vi "Read Log record configuration.vi"(8 "error in (no error)":errorcluster, 11 "Log Record in":refnum<class "Log Record.lvclass">) -> (0 "error out":errorcluster, 2 "Configuration":T1={"OSF node  ID"="", "Conection timeout"=60.0, "Station"="", "Log server "="magx", "Upload to OSF"=FALSE, "Append to lab book"=FALSE, "Filing modules"=["Monitor Controller", "Pulse Controller"]} {"Conection timeout" format="%#_6ps"}, 3 "Log Record out":refnum<class "Log Record.lvclass">)   [LabVIEW 2021, in "Log Record.lvclass"]
uses:
  Log Record.lvclass
  C:/GitHub/LabActor/Template Module/Template Module.lvclass
  Log Record Configuration.ctl
  Template Module/Template Module.lvclass/Template Module.ctl
  Template Module/Read Configuration.vi
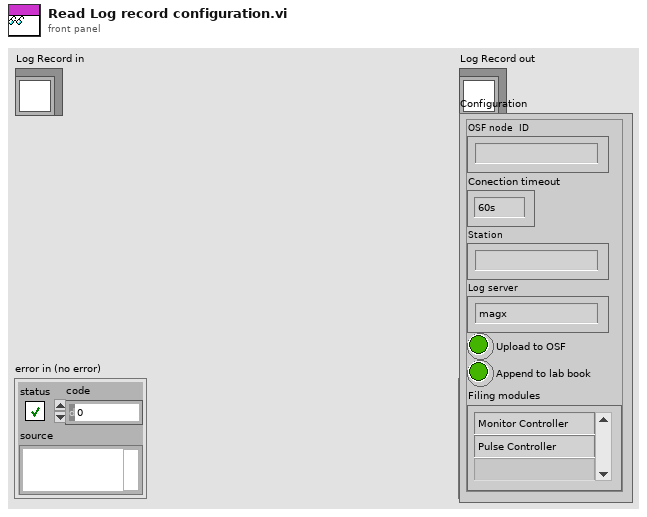
[diagram p1: front panel]
types:
  T1 = typedef "Log Record Configuration.ctl" = cluster{"OSF node  ID":string, "Conection timeout":dbl, "Station":string, "Log server ":string, "Upload to OSF":bool, "Append to lab book":bool, "Filing modules":string[]}
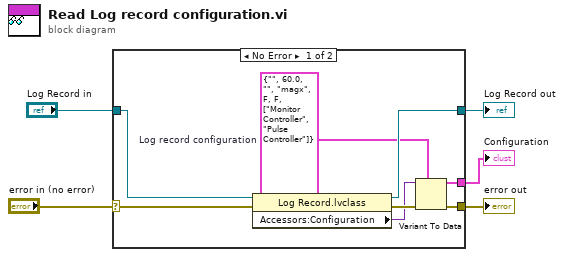
[diagram p0: block diagram]
diagram:
  n1 = case shown="No Error" "error in (no error)" {
    selector: "error in (no error)" -> [w13 w14]
    tunnel: [w9 w14] -> w4
    tunnel: [w10 w15] -> w2
    tunnel: "Log Record in" -> [w11 w15]
    tunnel: [w6 _] -> w1
    frame No Error {
      w8 = T1 {"OSF node  ID"="", "Conection timeout"=60.0, "Station"="", "Log server "="magx", "Upload to OSF"=FALSE, "Append to lab book"=FALSE, "Filing modules"=["Monitor Controller", "Pulse Controller"]}  # Log record configuration
      n2 = property class="Log Record.lvclass"(reference=w11, error in=w13) -> (reference out=w10:refnum<class "Log Record.lvclass">, error out=w12:errorcluster, "Accessors:Configuration"=w7:variant)
      n3 = Variant To Data(error in=w12, type=w8, Variant=w7) -> (data=w6:T1, error out=w9:errorcluster)
    }
    frame Error {
    }
  }
  "error out" <- w4
  "Log Record out" <- w2
  "Configuration" <- w1
